vi "sensor list attached sensors3.vi"(9 "dest_count":u32, 10 "buffer_length":u32, 11 "serial_number_buffer":u32) -> (1 "dest_count out":u32, 2 "function return":i32, 3 "serial_number_buffer out":u32)   [LabVIEW 2019, in "apdm.lvlib"]
doc: "APDM_EXPORT int apdm_sensor_list_attached_sensors3(uint32_t *serial_number_buffer, const uint32_t buffer_length, uint32_t *dest_count);"
uses:
  apdm.lvlib
  Lee Lab/CP FES Walking 2018/Code/Working/LabVIEW/apdm.dll
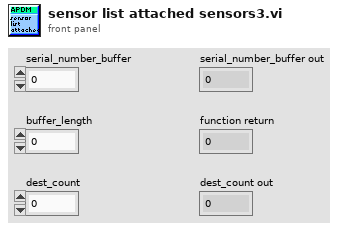
[diagram p1: front panel]
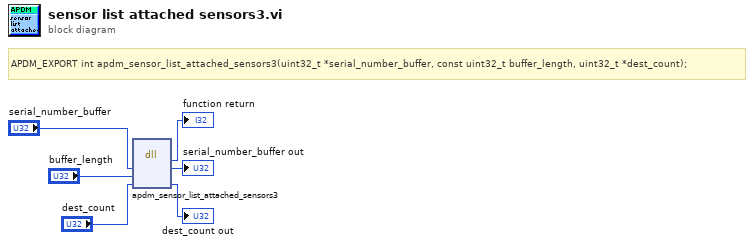
[diagram p0: block diagram]
diagram:
  # "APDM_EXPORT int apdm_sensor_list_attached_sensors3(uint32_t *serial_number_buffer, const uint32_t buffer_length, uint32_t *dest_count);"
  n1 = dll-call lib="C:/Users/jfalesi/Dropbox/Lee Lab/CP FES Walking 2018/Code/Working/LabVIEW/apdm.*" fn="apdm_sensor_list_attached_sensors3"("serial_number_buffer"="serial_number_buffer", "buffer_length"="buffer_length", "dest_count"="dest_count") -> (→"function return":i32, "serial_number_buffer"=→"serial_number_buffer out":u32, "dest_count"=→"dest_count out":u32)  [unwired: 4 in, 2 out]
